vi "parse_and_log_data.vi"(0 "Array":string[][](array[string]), 5 "Cluster":T1, 7 "file_log":bool=TRUE, 9 "log_num":i32, 11 "error in":errorcluster) -> (4 "Table 2":string[][](table), 6 "Num_out":i32, 15 "error out":errorcluster)   [LabVIEW 2023]
doc: "Used to parse and log data onto the given table and file."
uses:
  Controls/error_cluster.ctl
  Controls/errors_type.ctl
  <vilib>/Utility/error.llb/Trim Whitespace One-Sided.vi
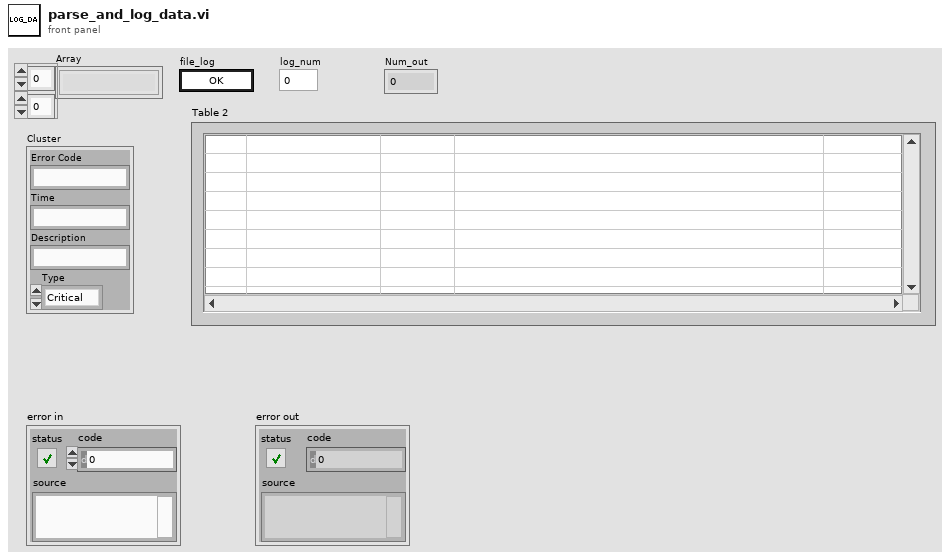
[diagram p1: front panel]
types:
  T1 = typedef "error_cluster.ctl" = cluster{"Error Code":string, "Time":string, "Description":string, "Type":T2}
  T2 = typedef "errors_type.ctl" = enum16{"Critical", "No error", "Warning", "Passive", "Unknown"}
  T3 = enum16{"open", "replace", "create", "open or create", "replace or create", "replace or create with confirmation"}
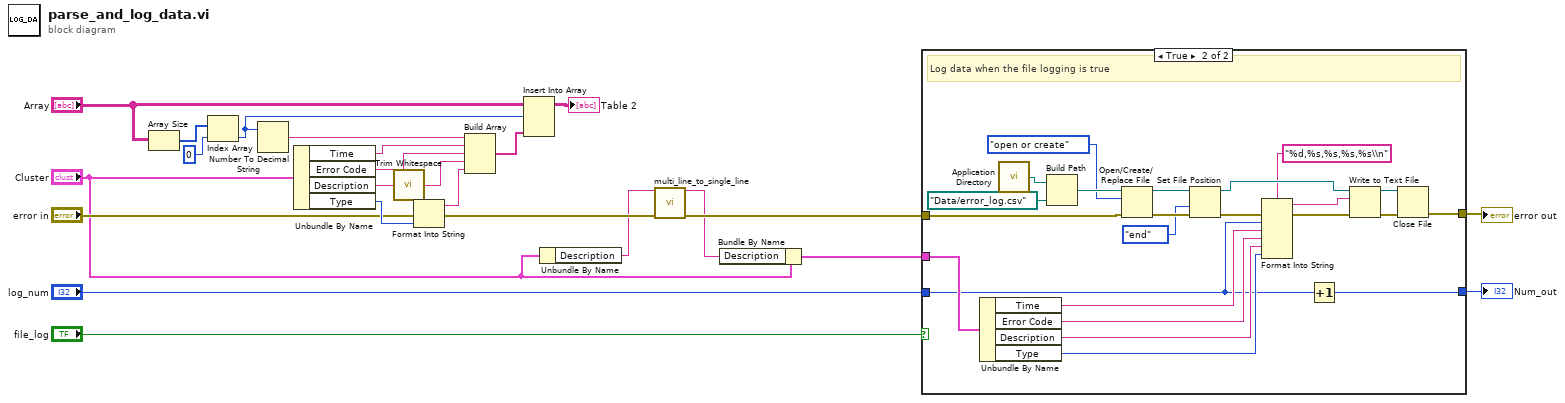
[diagram p0: block diagram]
diagram:
  n1 = Array Size(array="Array") -> (size(s)=w23:i32[])
  n2 = Index Array(array=w23, index=0) -> (element=w18:i32)
  n3 = Number To Decimal String(number=w18) -> (decimal integer string=w21:string)  [unwired: 1 in]
  n4 = Unbundle By Name("Cluster") -> ("Time"=w13:string, "Error Code"=w20:string, "Description"=w16:string, "Type"=w15:T2)
  n5 = call <vilib>:"Trim Whitespace.vi"("string"=w16) -> ("trimmed string"=w11:string)  [unwired: 1 in]
  n6 = Format Into String(error in="error in", w15) -> (resulting string=w14:string, error out=w4:errorcluster)  [unwired: 2 in]
  n7 = Build Array(w21, w13, w20, w11, w14) -> (w19:string[])
  n8 = Insert Into Array(array="Array", index (row)=w18, new element=w19) -> (→"Table 2":string[][])  [unwired: 1 in]
  n9 = Unbundle By Name("Cluster") -> ("Description"=w2:string)
  n10 = call "multi_line_to_single_line.vi"("input string"=w2, "error in (no error)"=w4) -> ("result string"=w1:string, "error out"=w3:errorcluster)  [unwired: 12 in]
  n11 = Bundle By Name(cluster="Cluster", "Description"=w1) -> (w6:T1)
  n12 = case shown="True" "file_log" {
    tunnel: w6 -> [_ w49]
    tunnel: w3 -> [w26 w45]
    tunnel: [w26 w39] -> w9
    tunnel: "log_num" -> [w25 w28]
    tunnel: [w25 w27] -> w7
    frame False {
      # "Does not log data onto file"
    }
    frame True {
      # "Log data when the file logging is true"
      n13 = Unbundle By Name(w49) -> ("Time"=w36:string, "Error Code"=w35:string, "Description"=w34:string, "Type"=w33:T2)
      n14 = call <vilib>:"Application Directory.vi"() -> ("Application Directory"=w48:path)
      n15 = Build Path(base path=w48, name or relative path=path "Data/error_log.csv") -> (appended path=w46:path)
      n16 = Open/Create/Replace File(file path (use dialog)=w46, error in=w45, operation (0:open)=T3."open or create") -> (refnum out=w41:refnum<file>, error out=w44:errorcluster)  [unwired: 3 in, 1 out]
      n17 = Set File Position(refnum=w41, from (0:start)=enum16{"start", "end", "current"}."end", error in=w44) -> (refnum out=w40:refnum<file>, error out=w31:errorcluster)  [unwired: 1 in]
      n18 = Format Into String(format string="%d,%s,%s,%s,%s\\n", error in=w31, w28, w36, w35, w34, w33) -> (resulting string=w32:string, error out=w30:errorcluster)  [unwired: 1 in]
      n19 = Increment(x=w28) -> (x+1=w27:i32)
      n20 = Write to Text File(file (use dialog)=w40, text=w32, error in=w30) -> (refnum out=w42:refnum<file>, error out=w43:errorcluster)  [unwired: 1 in, 1 out]
      n21 = Close File(refnum=w42, error in=w43) -> (error out=w39:errorcluster)  [unwired: 1 out]
    }
  }
  "error out" <- w9
  "Num_out" <- w7
